vi "Ic_FresnelLens.vi"(6 "Pixel Pitch 0:20um_or_ 1:12.5um":i32, 8 "error in (no error)":errorcluster, 9 "Wave length / nm":i32, 10 "Focus / mm":i32, 11 "2D array in (LCOS size buf)":u8[][](array[numeric])) -> (0 "error out":errorcluster, 3 "2D array out":u8[][](array[numeric]))   [LabVIEW 2013]
uses:
  SLM_Control_VI_source/Image_Control.dll
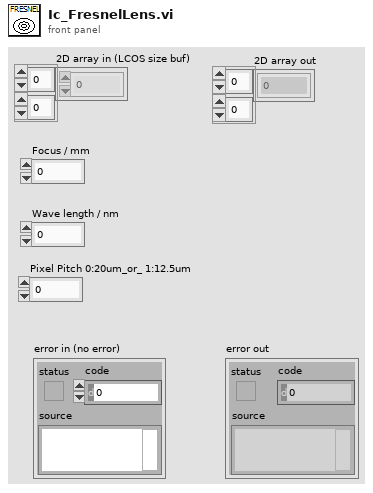
[diagram p1: front panel]
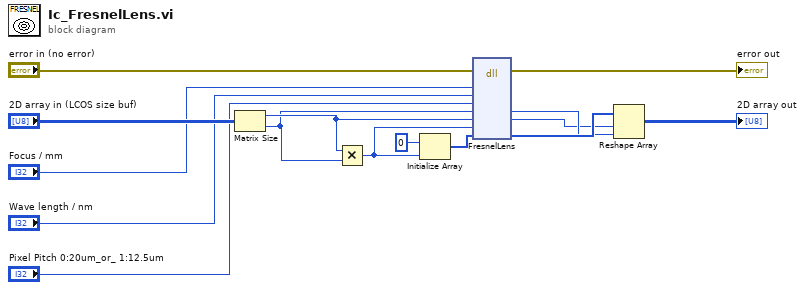
[diagram p0: block diagram]
diagram:
  n1 = Matrix Size(0:"2D array in (LCOS size buf)") -> (1:w2:i32, 2:w1:i32)
  n2 = Multiply(x=w2, y=w1) -> (x*y=w8:i32)
  n3 = Initialize Array(u8 0 ("要素"), w8) -> (w7:u8[])
  n4 = dll-call lib="C:/Users/hs5921/Desktop/SLM_Control_VI_source/Image_Control.dll" fn="FresnelLens"(error in="error in (no error)", "FocusMm"="Focus / mm", "WaveLengthNm"="Wave length / nm", "PixelPitch0:20um_or_1:12.5um"="Pixel Pitch 0:20um_or_ 1:12.5um", "X_pixel_target"=w1, "Y_pixel_target"=w2, "targetDataSize"=w8, "1DArrayOut"=w7) -> (error out=→"error out":errorcluster, "X_pixel_target"=w5:i32, "Y_pixel_target"=w4:i32, "1DArrayOut"=w6:u8[])  [unwired: 7 in, 1 out]
  n5 = Reshape Array(w6, w4, w5) -> (→"2D array out":u8[][])
